vi "Init.vi"(8 "error in":errorcluster, 11 "SimpleCsvDataLogger in":refnum<class "SimpleCsvDataLogger.lvclass">) -> (0 "error out":errorcluster, 3 "SimpleCsvDataLogger out":refnum<class "SimpleCsvDataLogger.lvclass">)   [LabVIEW 2019, in "SimpleCsvDataLogger.lvclass"]
uses:
  SimpleCsvDataLogger.lvclass
  SimpleCsvDataLogger.lvclass/SimpleCsvDataLogger.ctl
  Interfaces/IConfiguration/IConfiguration.lvclass
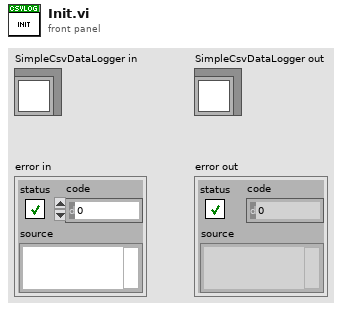
[diagram p1: front panel]
types:
  T1 = enum16{"open", "replace", "create", "open or create", "replace or create", "replace or create with confirmation"}
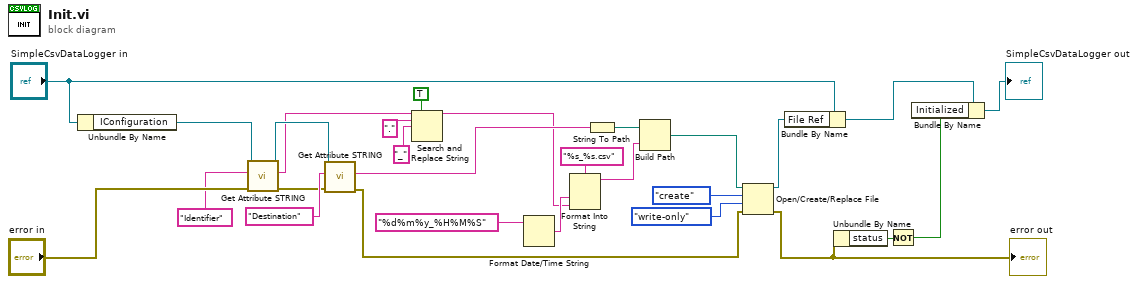
[diagram p0: block diagram]
diagram:
  n1 = Unbundle By Name("SimpleCsvDataLogger in") -> ("IConfiguration"=w27:refnum<class "IConfiguration.lvclass">)
  n2 = call-dynamic "Get Attribute STRING.vi"("error in"="error in", "Attribute"="Identifier", "IConfiguration in"=w27) -> ("error out"=w15:errorcluster, "Value"=w12:string, "IConfiguration out"=w17:refnum<class "IConfiguration.lvclass">)  [unwired: 6 in]
  n3 = call-dynamic "Get Attribute STRING.vi"("error in"=w15, "Attribute"="Destination", "IConfiguration in"=w17) -> ("error out"=w18:errorcluster, "Value"=w20:string)  [unwired: 6 in, 1 out]
  n4 = Search and Replace String(replace all?=TRUE ("replace all? (F)"), input string=w12, search string=".", replace string="_" ("replace string (\"\")")) -> (result string=w9:string)  [unwired: 4 in, 3 out]
  n5 = Format Date/Time String(time format string (%c)="%d%m%y_%H%M%S") -> (date/time string=w21:string)  [unwired: 2 in]
  n6 = Format Into String(format string="%s_%s.csv", w21, w9) -> (resulting string=w11:string)  [unwired: 2 in, 1 out]
  n7 = String To Path(string=w20) -> (path=w13:path)
  n8 = Build Path(base path=w13, name or relative path=w11) -> (appended path=w10:path)
  n9 = Open/Create/Replace File(file path (use dialog)=w10, error in=w18, operation (0:open)=T1."create", access (0:read/write)=enum16{"read/write", "read-only", "write-only"}."write-only") -> (refnum out=w19:refnum<file>, error out=w5:errorcluster)  [unwired: 2 in, 1 out]
  "error out" <- w5
  n10 = Bundle By Name(cluster="SimpleCsvDataLogger in", "File Ref"=w19) -> (w3:refnum<class "SimpleCsvDataLogger.lvclass">)
  n11 = Unbundle By Name(w5) -> ("status"=w4:bool)
  n12 = Not(x=w4) -> (.not. x?=w1:bool)
  n13 = Bundle By Name(cluster=w3, "Initialized"=w1) -> (→"SimpleCsvDataLogger out":refnum<class "SimpleCsvDataLogger.lvclass">)
